vi "LVClass_Pupil ctor from copy.vi"(0 "Pupil (const)":refnum<class "Pupil.lvclass">, 5 "Pupil to copy":refnum<class "Pupil.lvclass">, 11 "error constant":errorcluster) -> (4 "Pupil (new)":refnum<class "Pupil.lvclass">, 6 "Pupil to copy (dup)":refnum<class "Pupil.lvclass">, 15 "error IO":errorcluster)   [LabVIEW 2020, in "Pupil.lvclass"]
doc: "Circular Pupil constructor from dimensions, steps and circle shape.\n\n--------------------------------------------------------------------------------\n\n<B>PupilIn</B> : Constant Pointer to Pupil object.\n<B>PupilOut</B> : Pointer to Pupil object.\n<B>step</B> : Step x and y between the subpupils (um).\n<B>dimensions</B> : Pupil array dimensions (width, height).\n<B>center</B> : Center of the circle shape (um).\n<B>radius</B> : Radius of the circle shape (um).\n<B>ErrorIn</B> : Error\n<B>ErrorOut</B> : Error\n\n--------------------------------------------------------------------------------"
uses:
  Pupil.lvclass
  Controls/Handle creation.ctl
  Pupil.lvclass/Pupil.ctl
  LVClass_Pupil Read Pupil.vi
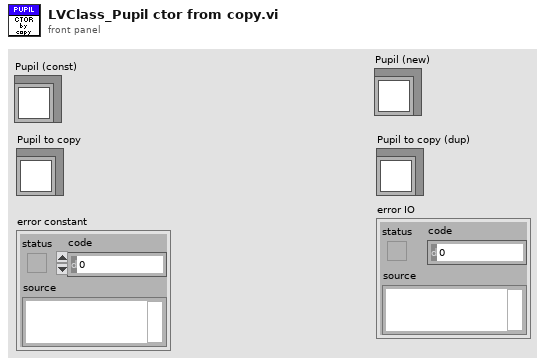
[diagram p1: front panel]
types:
  T1 = typedef "Handle creation.ctl" = enum16{"By ctor", "By write function"}
  T2 = typedef "ClassID.ctl" = i64
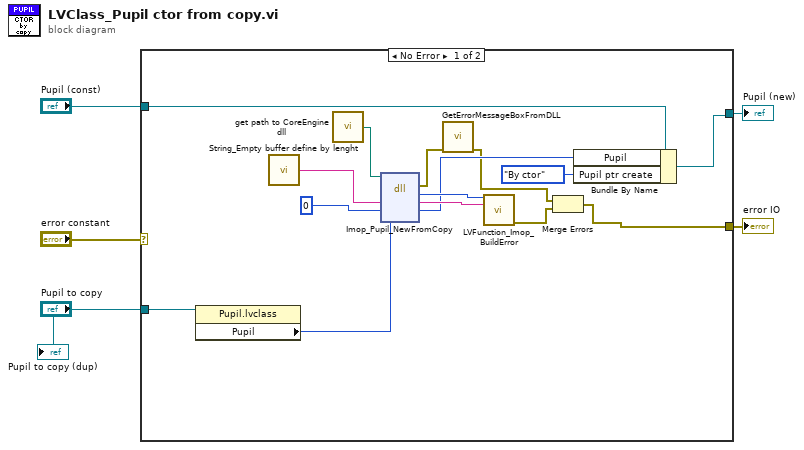
[diagram p0: block diagram]
diagram:
  n1 = case shown="No Error" "error constant" {
    selector: "error constant" -> [_ w22]
    tunnel: [w8 w22] -> w4
    tunnel: [w13 w21] -> w2
    tunnel: "Pupil (const)" -> [w14 w21]
    tunnel: "Pupil to copy" -> [w7 _]
    frame No Error {
      n2 = property class="Pupil.lvclass"(reference=w7) -> ("Pupil"=w6:T2)  [unwired: 1 in, 2 out]
      n3 = call "String_Empty buffer define by lenght.vi"() -> ("Empty buffer"=w20:string)  [unwired: 1 in]
      n4 = call "get path to CoreEngine dll.vi"() -> ("path to wavekit library"=w17:path)  [unwired: 14 in, 1 out]
      n5 = dll-call lib="D:/soft/HASO_v3/SVN_trunk/ImOpCoreEngine4_LV2011/DLLs/c_interface_vc100.dll" fn="Imop_Pupil_NewFromCopy"(path in=w17, "message"=w20, "Pupil"=0, "pupil_to_copy"=w6) -> (error out=w16:errorcluster, "return type"=w18:i32, "message"=w19:string, "Pupil"=w12:i64)  [unwired: 3 in, 1 out]
      n6 = call "GetErrorMessageBoxFromDLL.vi"("error IN"=w16) -> ("error OUT"=w10:errorcluster)  [unwired: 10 in]
      n7 = call "LVFunction_Imop_BuildError.vi"("code"=w18, "String to Prepend to source (\"\")"=w19) -> ("error out"=w9:errorcluster)  [unwired: 13 in]
      n8 = Merge Errors(w10, w9) -> (w8:errorcluster)
      n9 = Bundle By Name(cluster=w14, "Pupil"=w12, "Pupil ptr create"=Handle_creation."By ctor") -> (w13:refnum<class "Pupil.lvclass">)
    }
    frame Error {
    }
  }
  "error IO" <- w4
  "Pupil (new)" <- w2
  "Pupil to copy (dup)" <- "Pupil to copy"
